vi "OCV Histogram gRPC.vi"() -> (1 "mean values of channels":dbl[](array[numeric]), 2 "std dev":dbl, 3 "range":dbl)   [LabVIEW 2019] (continued)
  in  "OCVResults 200Hz":T1[](array[typedef])=[{"battery1voltage"=3.4816475, "battery2voltage"=3.4830532, "battery3voltage"=3.4783754, "battery4voltage"=3.4823782, "battery5voltage"=3.4844217, "battery6voltage"=0.0, "battery7voltage"=0.0, "battery8voltage"=0.0, "battery9voltage"=0.0, "battery10voltage"=0.0, "battery11voltage"=0.0, "battery12voltage"=0.0, "battery13voltage"=0.0, "battery14voltage"=0.0, "battery15voltage"=0.0, "battery16voltage"=0.0, "battery17voltage"=0.0, "battery18voltage"=0.0, "battery19voltage"=0.0, "battery20voltage"=0.0, "battery21voltage"=0.0, "battery22voltage"=0.0, "battery23voltage"=0.0, "battery24voltage"=0.0, "ErrorOutData"={"ErrorCode"=0, "ErrorMessage"=""}}, {"battery1voltage"=3.4816465, "battery2voltage"=3.4830518, "battery3voltage"=3.4783754, "battery4voltage"=3.4823792, "battery5voltage"=3.484419, "battery6voltage"=0.0, "battery7voltage"=0.0, "battery8voltage"=0.0, "battery9voltage"=0.0, "battery10voltage"=0.0, "battery11voltage"=0.0, "battery12voltage"=0.0, "battery13voltage"=0.0, "battery14voltage"=0.0, "battery15voltage"=0.0, "battery16voltage"=0.0, "battery17voltage"=0.0, "battery18voltage"=0.0, "battery19voltage"=0.0, "battery20voltage"=0.0, "battery21voltage"=0.0, "battery22voltage"=0.0, "battery23voltage"=0.0, "battery24voltage"=0.0, "ErrorOutData"={"ErrorCode"=0, "ErrorMessage"=""}}, {"battery1voltage"=3.4816508, "battery2voltage"=3.483053, "battery3voltage"=3.4783792, "battery4voltage"=3.482379, "battery5voltage"=3.484414, "battery6voltage"=0.0, "battery7voltage"=0.0, "battery8voltage"=0.0, "battery9voltage"=0.0, "battery10voltage"=0.0, "battery11voltage"=0.0, "battery12voltage"=0.0, "battery13voltage"=0.0, "battery14voltage"=0.0, "battery15voltage"=0.0, "battery16voltage"=0.0, "battery17voltage"=0.0, "battery18voltage"=0.0, "battery19voltage"=0.0, "battery20voltage"=0.0, "battery21voltage"=0.0, "battery22voltage"=0.0, "battery23voltage"=0.0, "battery24voltage"=0.0, "ErrorOutData"={"ErrorCode"=0, "ErrorMessage"=""}}, {"battery1voltage"=3.4816496, "battery2voltage"=3.4830558, "battery3voltage"=3.4783785, "battery4voltage"=3.4823782, "battery5voltage"=3.484414, "battery6voltage"=0.0, "battery7voltage"=0.0, "battery8voltage"=0.0, "battery9voltage"=0.0, "battery10voltage"=0.0, "battery11voltage"=0.0, "battery12voltage"=0.0, "battery13voltage"=0.0, "battery14voltage"=0.0, "battery15voltage"=0.0, "battery16voltage"=0.0, "battery17voltage"=0.0, "battery18voltage"=0.0, "battery19voltage"=0.0, "battery20voltage"=0.0, "battery21voltage"=0.0, "battery22voltage"=0.0, "battery23voltage"=0.0, "battery24voltage"=0.0, "ErrorOutData"={"ErrorCode"=0, "ErrorMessage"=""}}, {"battery1voltage"=3.481646, "battery2voltage"=3.4830523, "battery3voltage"=3.4783762, "battery4voltage"=3.482376, "battery5voltage"=3.4844196, "battery6voltage"=0.0, "battery7voltage"=0.0, "battery8voltage"=0.0, "battery9voltage"=0.0, "battery10voltage"=0.0, "battery11voltage"=0.0, "battery12voltage"=0.0, "battery13voltage"=0.0, "battery14voltage"=0.0, "battery15voltage"=0.0, "battery16voltage"=0.0, "battery17voltage"=0.0, "battery18voltage"=0.0, "battery19voltage"=0.0, "battery20voltage"=0.0, "battery21voltage"=0.0, "battery22voltage"=0.0, "battery23voltage"=0.0, "battery24voltage"=0.0, "ErrorOutData"={"ErrorCode"=0, "ErrorMessage"=""}}, {"battery1voltage"=3.481651, "battery2voltage"=3.4830537, "battery3voltage"=3.4783807, "battery4voltage"=3.4823775, "battery5voltage"=3.484415, "battery6voltage"=0.0, "battery7voltage"=0.0, "battery8voltage"=0.0, "battery9voltage"=0.0, "battery10voltage"=0.0, "battery11voltage"=0.0, "battery12voltage"=0.0, "battery13voltage"=0.0, "battery14voltage"=0.0, "battery15voltage"=0.0, "battery16voltage"=0.0, "battery17voltage"=0.0, "battery18voltage"=0.0, "battery19voltage"=0.0, "battery20voltage"=0.0, "battery21voltage"=0.0, "battery22voltage"=0.0, "battery23voltage"=0.0, "battery24voltage"=0.0, "ErrorOutData"={"ErrorCode"=0, "ErrorMessage"=""}}, {"battery1voltage"=3.4816496, "battery2voltage"=3.4830575, "battery3voltage"=3.4783802, "battery4voltage"=3.4823804, "battery5voltage"=3.4844165, "battery6voltage"=0.0, "battery7voltage"=0.0, "battery8voltage"=0.0, "battery9voltage"=0.0, "battery10voltage"=0.0, "battery11voltage"=0.0, "battery12voltage"=0.0, "battery13voltage"=0.0, "battery14voltage"=0.0, "battery15voltage"=0.0, "battery16voltage"=0.0, "battery17voltage"=0.0, "battery18voltage"=0.0, "battery19voltage"=0.0, "battery20voltage"=0.0, "battery21voltage"=0.0, "battery22voltage"=0.0, "battery23voltage"=0.0, "battery24voltage"=0.0, "ErrorOutData"={"ErrorCode"=0, "ErrorMessage"=""}}, {"battery1voltage"=3.4816468, "battery2voltage"=3.4830506, "battery3voltage"=3.4783757, "battery4voltage"=3.4823778, "battery5voltage"=3.484419, "battery6voltage"=0.0, "battery7voltage"=0.0, "battery8voltage"=0.0, "battery9voltage"=0.0, "battery10voltage"=0.0, "battery11voltage"=0.0, "battery12voltage"=0.0, "battery13voltage"=0.0, "battery14voltage"=0.0, "battery15voltage"=0.0, "battery16voltage"=0.0, "battery17voltage"=0.0, "battery18voltage"=0.0, "battery19voltage"=0.0, "battery20voltage"=0.0, "battery21voltage"=0.0, "battery22voltage"=0.0, "battery23voltage"=0.0, "battery24voltage"=0.0, "ErrorOutData"={"ErrorCode"=0, "ErrorMessage"=""}}, {"battery1voltage"=3.4816494, "battery2voltage"=3.4830542, "battery3voltage"=3.4783788, "battery4voltage"=3.4823797, "battery5voltage"=3.4844136, "battery6voltage"=0.0, "battery7voltage"=0.0, "battery8voltage"=0.0, "battery9voltage"=0.0, "battery10voltage"=0.0, "battery11voltage"=0.0, "battery12voltage"=0.0, "battery13voltage"=0.0, "battery14voltage"=0.0, "battery15voltage"=0.0, "battery16voltage"=0.0, "battery17voltage"=0.0, "battery18voltage"=0.0, "battery19voltage"=0.0, "battery20voltage"=0.0, "battery21voltage"=0.0, "battery22voltage"=0.0, "battery23voltage"=0.0, "battery24voltage"=0.0, "ErrorOutData"={"ErrorCode"=0, "ErrorMessage"=""}}, {"battery1voltage"=3.4816506, "battery2voltage"=3.483054, "battery3voltage"=3.4783807, "battery4voltage"=3.4823804, "battery5voltage"=3.4844153, "battery6voltage"=0.0, "battery7voltage"=0.0, "battery8voltage"=0.0, "battery9voltage"=0.0, "battery10voltage"=0.0, "battery11voltage"=0.0, "battery12voltage"=0.0, "battery13voltage"=0.0, "battery14voltage"=0.0, "battery15voltage"=0.0, "battery16voltage"=0.0, "battery17voltage"=0.0, "battery18voltage"=0.0, "battery19voltage"=0.0, "battery20voltage"=0.0, "battery21voltage"=0.0, "battery22voltage"=0.0, "battery23voltage"=0.0, "battery24voltage"=0.0, "ErrorOutData"={"ErrorCode"=0, "ErrorMessage"=""}}, {"battery1voltage"=3.481649, "battery2voltage"=3.4830494, "battery3voltage"=3.478376, "battery4voltage"=3.482376, "battery5voltage"=3.4844186, "battery6voltage"=0.0, "battery7voltage"=0.0, "battery8voltage"=0.0, "battery9voltage"=0.0, "battery10voltage"=0.0, "battery11voltage"=0.0, "battery12voltage"=0.0, "battery13voltage"=0.0, "battery14voltage"=0.0, "battery15voltage"=0.0, "battery16voltage"=0.0, "battery17voltage"=0.0, "battery18voltage"=0.0, "battery19voltage"=0.0, "battery20voltage"=0.0, "battery21voltage"=0.0, "battery22voltage"=0.0, "battery23voltage"=0.0, "battery24voltage"=0.0, "ErrorOutData"={"ErrorCode"=0, "ErrorMessage"=""}}, {"battery1voltage"=3.4816506, "battery2voltage"=3.483054, "battery3voltage"=3.4783802, "battery4voltage"=3.4823794, "battery5voltage"=3.4844139, "battery6voltage"=0.0, "battery7voltage"=0.0, "battery8voltage"=0.0, "battery9voltage"=0.0, "battery10voltage"=0.0, "battery11voltage"=0.0, "battery12voltage"=0.0, "battery13voltage"=0.0, "battery14voltage"=0.0, "battery15voltage"=0.0, "battery16voltage"=0.0, "battery17voltage"=0.0, "battery18voltage"=0.0, "battery19voltage"=0.0, "battery20voltage"=0.0, "battery21voltage"=0.0, "battery22voltage"=0.0, "battery23voltage"=0.0, "battery24voltage"=0.0, "ErrorOutData"={"ErrorCode"=0, "ErrorMessage"=""}}, {"battery1voltage"=3.481648, "battery2voltage"=3.483055, "battery3voltage"=3.4783783, "battery4voltage"=3.482379, "battery5voltage"=3.484413, "battery6voltage"=0.0, "battery7voltage"=0.0, "battery8voltage"=0.0, "battery9voltage"=0.0, "battery10voltage"=0.0, "battery11voltage"=0.0, "battery12voltage"=0.0, "battery13voltage"=0.0, "battery14voltage"=0.0, "battery15voltage"=0.0, "battery16voltage"=0.0, "battery17voltage"=0.0, "battery18voltage"=0.0, "battery19voltage"=0.0, "battery20voltage"=0.0, "battery21voltage"=0.0, "battery22voltage"=0.0, "battery23voltage"=0.0, "battery24voltage"=0.0, "ErrorOutData"={"ErrorCode"=0, "ErrorMessage"=""}}, {"battery1voltage"=3.4816458, "battery2voltage"=3.483052, "battery3voltage"=3.4783766, "battery4voltage"=3.4823794, "battery5voltage"=3.484419, "battery6voltage"=0.0, "battery7voltage"=0.0, "battery8voltage"=0.0, "battery9voltage"=0.0, "battery10voltage"=0.0, "battery11voltage"=0.0, "battery12voltage"=0.0, "battery13voltage"=0.0, "battery14voltage"=0.0, "battery15voltage"=0.0, "battery16voltage"=0.0, "battery17voltage"=0.0, "battery18voltage"=0.0, "battery19voltage"=0.0, "battery20voltage"=0.0, "battery21voltage"=0.0, "battery22voltage"=0.0, "battery23voltage"=0.0, "battery24voltage"=0.0, "ErrorOutData"={"ErrorCode"=0, "ErrorMessage"=""}}, {"battery1voltage"=3.4816475, "battery2voltage"=3.4830542, "battery3voltage"=3.4783762, "battery4voltage"=3.482376, "battery5voltage"=3.484421, "battery6voltage"=0.0, "battery7voltage"=0.0, "battery8voltage"=0.0, "battery9voltage"=0.0, "battery10voltage"=0.0, "battery11voltage"=0.0, "battery12voltage"=0.0, "battery13voltage"=0.0, "battery14voltage"=0.0, "battery15voltage"=0.0, "battery16voltage"=0.0, "battery17voltage"=0.0, "battery18voltage"=0.0, "battery19voltage"=0.0, "battery20voltage"=0.0, "battery21voltage"=0.0, "battery22voltage"=0.0, "battery23voltage"=0.0, "battery24voltage"=0.0, "ErrorOutData"={"ErrorCode"=0, "ErrorMessage"=""}}, {"battery1voltage"=3.4816487, "battery2voltage"=3.4830506, "battery3voltage"=3.4783754, "battery4voltage"=3.482377, "battery5voltage"=3.4844167, "battery6voltage"=0.0, "battery7voltage"=0.0, "battery8voltage"=0.0, "battery9voltage"=0.0, "battery10voltage"=0.0, "battery11voltage"=0.0, "battery12voltage"=0.0, "battery13voltage"=0.0, "battery14voltage"=0.0, "battery15voltage"=0.0, "battery16voltage"=0.0, "battery17voltage"=0.0, "battery18voltage"=0.0, "battery19voltage"=0.0, "battery20voltage"=0.0, "battery21voltage"=0.0, "battery22voltage"=0.0, "battery23voltage"=0.0, "battery24voltage"=0.0, "ErrorOutData"={"ErrorCode"=0, "ErrorMessage"=""}}, {"battery1voltage"=3.4816504, "battery2voltage"=3.483053, "battery3voltage"=3.4783785, "battery4voltage"=3.4823782, "battery5voltage"=3.4844148, "battery6voltage"=0.0, "battery7voltage"=0.0, "battery8voltage"=0.0, "battery9voltage"=0.0, "battery10voltage"=0.0, "battery11voltage"=0.0, "battery12voltage"=0.0, "battery13voltage"=0.0, "battery14voltage"=0.0, "battery15voltage"=0.0, "battery16voltage"=0.0, "battery17voltage"=0.0, "battery18voltage"=0.0, "battery19voltage"=0.0, "battery20voltage"=0.0, "battery21voltage"=0.0, "battery22voltage"=0.0, "battery23voltage"=0.0, "battery24voltage"=0.0, "ErrorOutData"={"ErrorCode"=0, "ErrorMessage"=""}}, {"battery1voltage"=3.4816487, "battery2voltage"=3.4830518, "battery3voltage"=3.4783754, "battery4voltage"=3.482377, "battery5voltage"=3.4844203, "battery6voltage"=0.0, "battery7voltage"=0.0, "battery8voltage"=0.0, "battery9voltage"=0.0, "battery10voltage"=0.0, "battery11voltage"=0.0, "battery12voltage"=0.0, "battery13voltage"=0.0, "battery14voltage"=0.0, "battery15voltage"=0.0, "battery16voltage"=0.0, "battery17voltage"=0.0, "battery18voltage"=0.0, "battery19voltage"=0.0, "battery20voltage"=0.0, "battery21voltage"=0.0, "battery22voltage"=0.0, "battery23voltage"=0.0, "battery24voltage"=0.0, "ErrorOutData"={"ErrorCode"=0, "ErrorMessage"=""}}, {"battery1voltage"=3.4816482, "battery2voltage"=3.4830515, "battery3voltage"=3.4783762, "battery4voltage"=3.4823794, "battery5voltage"=3.484422, "battery6voltage"=0.0, "battery7voltage"=0.0, "battery8voltage"=0.0, "battery9voltage"=0.0, "battery10voltage"=0.0, "battery11voltage"=0.0, "battery12voltage"=0.0, "battery13voltage"=0.0, "battery14voltage"=0.0, "battery15voltage"=0.0, "battery16voltage"=0.0, "battery17voltage"=0.0, "battery18voltage"=0.0, "battery19voltage"=0.0, "battery20voltage"=0.0, "battery21voltage"=0.0, "battery22voltage"=0.0, "battery23voltage"=0.0, "battery24voltage"=0.0, "ErrorOutData"={"ErrorCode"=0, "ErrorMessage"=""}}, {"battery1voltage"=3.4816468, "battery2voltage"=3.4830506, "battery3voltage"=3.478376, "battery4voltage"=3.4823782, "battery5voltage"=3.484421, "battery6voltage"=0.0, "battery7voltage"=0.0, "battery8voltage"=0.0, "battery9voltage"=0.0, "battery10voltage"=0.0, "battery11voltage"=0.0, "battery12voltage"=0.0, "battery13voltage"=0.0, "battery14voltage"=0.0, "battery15voltage"=0.0, "battery16voltage"=0.0, "battery17voltage"=0.0, "battery18voltage"=0.0, "battery19voltage"=0.0, "battery20voltage"=0.0, "battery21voltage"=0.0, "battery22voltage"=0.0, "battery23voltage"=0.0, "battery24voltage"=0.0, "ErrorOutData"={"ErrorCode"=0, "ErrorMessage"=""}}, {"battery1voltage"=3.4816484, "battery2voltage"=3.4830525, "battery3voltage"=3.4783764, "battery4voltage"=3.4823756, "battery5voltage"=3.4844203, "battery6voltage"=0.0, "battery7voltage"=0.0, "battery8voltage"=0.0, "battery9voltage"=0.0, "battery10voltage"=0.0, "battery11voltage"=0.0, "battery12voltage"=0.0, "battery13voltage"=0.0, "battery14voltage"=0.0, "battery15voltage"=0.0, "battery16voltage"=0.0, "battery17voltage"=0.0, "battery18voltage"=0.0, "battery19voltage"=0.0, "battery20voltage"=0.0, "battery21voltage"=0.0, "battery22voltage"=0.0, "battery23voltage"=0.0, "battery24voltage"=0.0, "ErrorOutData"={"ErrorCode"=0, "ErrorMessage"=""}}, {"battery1voltage"=3.4816477, "battery2voltage"=3.4830525, "battery3voltage"=3.4783745, "battery4voltage"=3.482378, "battery5voltage"=3.484421, "battery6voltage"=0.0, "battery7voltage"=0.0, "battery8voltage"=0.0, "battery9voltage"=0.0, "battery10voltage"=0.0, "battery11voltage"=0.0, "battery12voltage"=0.0, "battery13voltage"=0.0, "battery14voltage"=0.0, "battery15voltage"=0.0, "battery16voltage"=0.0, "battery17voltage"=0.0, "battery18voltage"=0.0, "battery19voltage"=0.0, "battery20voltage"=0.0, "battery21voltage"=0.0, "battery22voltage"=0.0, "battery23voltage"=0.0, "battery24voltage"=0.0, "ErrorOutData"={"ErrorCode"=0, "ErrorMessage"=""}}, {"battery1voltage"=3.4816477, "battery2voltage"=3.4830518, "battery3voltage"=3.4783752, "battery4voltage"=3.4823785, "battery5voltage"=3.4844203, "battery6voltage"=0.0, "battery7voltage"=0.0, "battery8voltage"=0.0, "battery9voltage"=0.0, "battery10voltage"=0.0, "battery11voltage"=0.0, "battery12voltage"=0.0, "battery13voltage"=0.0, "battery14voltage"=0.0, "battery15voltage"=0.0, "battery16voltage"=0.0, "battery17voltage"=0.0, "battery18voltage"=0.0, "battery19voltage"=0.0, "battery20voltage"=0.0, "battery21voltage"=0.0, "battery22voltage"=0.0, "battery23voltage"=0.0, "battery24voltage"=0.0, "ErrorOutData"={"ErrorCode"=0, "ErrorMessage"=""}}, {"battery1voltage"=3.4816518, "battery2voltage"=3.4830563, "battery3voltage"=3.47838, "battery4voltage"=3.4823773, "battery5voltage"=3.4844139, "battery6voltage"=0.0, "battery7voltage"=0.0, "battery8voltage"=0.0, "battery9voltage"=0.0, "battery10voltage"=0.0, "battery11voltage"=0.0, "battery12voltage"=0.0, "battery13voltage"=0.0, "battery14voltage"=0.0, "battery15voltage"=0.0, "battery16voltage"=0.0, "battery17voltage"=0.0, "battery18voltage"=0.0, "battery19voltage"=0.0, "battery20voltage"=0.0, "battery21voltage"=0.0, "battery22voltage"=0.0, "battery23voltage"=0.0, "battery24voltage"=0.0, "ErrorOutData"={"ErrorCode"=0, "ErrorMessage"=""}}, {"battery1voltage"=3.4816487, "battery2voltage"=3.483055, "battery3voltage"=3.478379, "battery4voltage"=3.4823766, "battery5voltage"=3.484415, "battery6voltage"=0.0, "battery7voltage"=0.0, "battery8voltage"=0.0, "battery9voltage"=0.0, "battery10voltage"=0.0, "battery11voltage"=0.0, "battery12voltage"=0.0, "battery13voltage"=0.0, "battery14voltage"=0.0, "battery15voltage"=0.0, "battery16voltage"=0.0, "battery17voltage"=0.0, "battery18voltage"=0.0, "battery19voltage"=0.0, "battery20voltage"=0.0, "battery21voltage"=0.0, "battery22voltage"=0.0, "battery23voltage"=0.0, "battery24voltage"=0.0, "ErrorOutData"={"ErrorCode"=0, "ErrorMessage"=""}}, {"battery1voltage"=3.4816518, "battery2voltage"=3.483055, "battery3voltage"=3.4783797, "battery4voltage"=3.4823785, "battery5voltage"=3.4844165, "battery6voltage"=0.0, "battery7voltage"=0.0, "battery8voltage"=0.0, "battery9voltage"=0.0, "battery10voltage"=0.0, "battery11voltage"=0.0, "battery12voltage"=0.0, "battery13voltage"=0.0, "battery14voltage"=0.0, "battery15voltage"=0.0, "battery16voltage"=0.0, "battery17voltage"=0.0, "battery18voltage"=0.0, "battery19voltage"=0.0, "battery20voltage"=0.0, "battery21voltage"=0.0, "battery22voltage"=0.0, "battery23voltage"=0.0, "battery24voltage"=0.0, "ErrorOutData"={"ErrorCode"=0, "ErrorMessage"=""}}, {"battery1voltage"=3.481648, "battery2voltage"=3.4830523, "battery3voltage"=3.4783738, "battery4voltage"=3.4823773, "battery5voltage"=3.48442, "battery6voltage"=0.0, "battery7voltage"=0.0, "battery8voltage"=0.0, "battery9voltage"=0.0, "battery10voltage"=0.0, "battery11voltage"=0.0, "battery12voltage"=0.0, "battery13voltage"=0.0, "battery14voltage"=0.0, "battery15voltage"=0.0, "battery16voltage"=0.0, "battery17voltage"=0.0, "battery18voltage"=0.0, "battery19voltage"=0.0, "battery20voltage"=0.0, "battery21voltage"=0.0, "battery22voltage"=0.0, "battery23voltage"=0.0, "battery24voltage"=0.0, "ErrorOutData"={"ErrorCode"=0, "ErrorMessage"=""}}, {"battery1voltage"=3.481649, "battery2voltage"=3.4830487, "battery3voltage"=3.4783742, "battery4voltage"=3.482377, "battery5voltage"=3.484417, "battery6voltage"=0.0, "battery7voltage"=0.0, "battery8voltage"=0.0, "battery9voltage"=0.0, "battery10voltage"=0.0, "battery11voltage"=0.0, "battery12voltage"=0.0, "battery13voltage"=0.0, "battery14voltage"=0.0, "battery15voltage"=0.0, "battery16voltage"=0.0, "battery17voltage"=0.0, "battery18voltage"=0.0, "battery19voltage"=0.0, "battery20voltage"=0.0, "battery21voltage"=0.0, "battery22voltage"=0.0, "battery23voltage"=0.0, "battery24voltage"=0.0, "ErrorOutData"={"ErrorCode"=0, "ErrorMessage"=""}}, {"battery1voltage"=3.4816473, "battery2voltage"=3.4830534, "battery3voltage"=3.4783776, "battery4voltage"=3.4823763, "battery5voltage"=3.4844205, "battery6voltage"=0.0, "battery7voltage"=0.0, "battery8voltage"=0.0, "battery9voltage"=0.0, "battery10voltage"=0.0, "battery11voltage"=0.0, "battery12voltage"=0.0, "battery13voltage"=0.0, "battery14voltage"=0.0, "battery15voltage"=0.0, "battery16voltage"=0.0, "battery17voltage"=0.0, "battery18voltage"=0.0, "battery19voltage"=0.0, "battery20voltage"=0.0, "battery21voltage"=0.0, "battery22voltage"=0.0, "battery23voltage"=0.0, "battery24voltage"=0.0, "ErrorOutData"={"ErrorCode"=0, "ErrorMessage"=""}}, {"battery1voltage"=3.4816482, "battery2voltage"=3.4830527, "battery3voltage"=3.4783754, "battery4voltage"=3.482379, "battery5voltage"=3.4844193, "battery6voltage"=0.0, "battery7voltage"=0.0, "battery8voltage"=0.0, "battery9voltage"=0.0, "battery10voltage"=0.0, "battery11voltage"=0.0, "battery12voltage"=0.0, "battery13voltage"=0.0, "battery14voltage"=0.0, "battery15voltage"=0.0, "battery16voltage"=0.0, "battery17voltage"=0.0, "battery18voltage"=0.0, "battery19voltage"=0.0, "battery20voltage"=0.0, "battery21voltage"=0.0, "battery22voltage"=0.0, "battery23voltage"=0.0, "battery24voltage"=0.0, "ErrorOutData"={"ErrorCode"=0, "ErrorMessage"=""}}, {"battery1voltage"=3.4816475, "battery2voltage"=3.4830527, "battery3voltage"=3.4783762, "battery4voltage"=3.4823744, "battery5voltage"=3.4844196, "battery6voltage"=0.0, "battery7voltage"=0.0, "battery8voltage"=0.0, "battery9voltage"=0.0, "battery10voltage"=0.0, "battery11voltage"=0.0, "battery12voltage"=0.0, "battery13voltage"=0.0, "battery14voltage"=0.0, "battery15voltage"=0.0, "battery16voltage"=0.0, "battery17voltage"=0.0, "battery18voltage"=0.0, "battery19voltage"=0.0, "battery20voltage"=0.0, "battery21voltage"=0.0, "battery22voltage"=0.0, "battery23voltage"=0.0, "battery24voltage"=0.0, "ErrorOutData"={"ErrorCode"=0, "ErrorMessage"=""}}, {"battery1voltage"=3.4816487, "battery2voltage"=3.4830544, "battery3voltage"=3.478379, "battery4voltage"=3.4823763, "battery5voltage"=3.4844158, "battery6voltage"=0.0, "battery7voltage"=0.0, "battery8voltage"=0.0, "battery9voltage"=0.0, "battery10voltage"=0.0, "battery11voltage"=0.0, "battery12voltage"=0.0, "battery13voltage"=0.0, "battery14voltage"=0.0, "battery15voltage"=0.0, "battery16voltage"=0.0, "battery17voltage"=0.0, "battery18voltage"=0.0, "battery19voltage"=0.0, "battery20voltage"=0.0, "battery21voltage"=0.0, "battery22voltage"=0.0, "battery23voltage"=0.0, "battery24voltage"=0.0, "ErrorOutData"={"ErrorCode"=0, "ErrorMessage"=""}}, {"battery1voltage"=3.481652, "battery2voltage"=3.4830534, "battery3voltage"=3.4783797, "battery4voltage"=3.4823794, "battery5voltage"=3.4844155, "battery6voltage"=0.0, "battery7voltage"=0.0, "battery8voltage"=0.0, "battery9voltage"=0.0, "battery10voltage"=0.0, "battery11voltage"=0.0, "battery12voltage"=0.0, "battery13voltage"=0.0, "battery14voltage"=0.0, "battery15voltage"=0.0, "battery16voltage"=0.0, "battery17voltage"=0.0, "battery18voltage"=0.0, "battery19voltage"=0.0, "battery20voltage"=0.0, "battery21voltage"=0.0, "battery22voltage"=0.0, "battery23voltage"=0.0, "battery24voltage"=0.0, "ErrorOutData"={"ErrorCode"=0, "ErrorMessage"=""}}, {"battery1voltage"=3.481647, "battery2voltage"=3.483051, "battery3voltage"=3.4783762, "battery4voltage"=3.4823768, "battery5voltage"=3.4844208, "battery6voltage"=0.0, "battery7voltage"=0.0, "battery8voltage"=0.0, "battery9voltage"=0.0, "battery10voltage"=0.0, "battery11voltage"=0.0, "battery12voltage"=0.0, "battery13voltage"=0.0, "battery14voltage"=0.0, "battery15voltage"=0.0, "battery16voltage"=0.0, "battery17voltage"=0.0, "battery18voltage"=0.0, "battery19voltage"=0.0, "battery20voltage"=0.0, "battery21voltage"=0.0, "battery22voltage"=0.0, "battery23voltage"=0.0, "battery24voltage"=0.0, "ErrorOutData"={"ErrorCode"=0, "ErrorMessage"=""}}, {"battery1voltage"=3.481646, "battery2voltage"=3.4830496, "battery3voltage"=3.4783783, "battery4voltage"=3.4823778, "battery5voltage"=3.4844189, "battery6voltage"=0.0, "battery7voltage"=0.0, "battery8voltage"=0.0, "battery9voltage"=0.0, "battery10voltage"=0.0, "battery11voltage"=0.0, "battery12voltage"=0.0, "battery13voltage"=0.0, "battery14voltage"=0.0, "battery15voltage"=0.0, "battery16voltage"=0.0, "battery17voltage"=0.0, "battery18voltage"=0.0, "battery19voltage"=0.0, "battery20voltage"=0.0, "battery21voltage"=0.0, "battery22voltage"=0.0, "battery23voltage"=0.0, "battery24voltage"=0.0, "ErrorOutData"={"ErrorCode"=0, "ErrorMessage"=""}}, {"battery1voltage"=3.4816482, "battery2voltage"=3.4830515, "battery3voltage"=3.4783747, "battery4voltage"=3.4823802, "battery5voltage"=3.484419, "battery6voltage"=0.0, "battery7voltage"=0.0, "battery8voltage"=0.0, "battery9voltage"=0.0, "battery10voltage"=0.0, "battery11voltage"=0.0, "battery12voltage"=0.0, "battery13voltage"=0.0, "battery14voltage"=0.0, "battery15voltage"=0.0, "battery16voltage"=0.0, "battery17voltage"=0.0, "battery18voltage"=0.0, "battery19voltage"=0.0, "battery20voltage"=0.0, "battery21voltage"=0.0, "battery22voltage"=0.0, "battery23voltage"=0.0, "battery24voltage"=0.0, "ErrorOutData"={"ErrorCode"=0, "ErrorMessage"=""}}, {"battery1voltage"=3.4816465, "battery2voltage"=3.48305, "battery3voltage"=3.4783783, "battery4voltage"=3.4823782, "battery5voltage"=3.4844184, "battery6voltage"=0.0, "battery7voltage"=0.0, "battery8voltage"=0.0, "battery9voltage"=0.0, "battery10voltage"=0.0, "battery11voltage"=0.0, "battery12voltage"=0.0, "battery13voltage"=0.0, "battery14voltage"=0.0, "battery15voltage"=0.0, "battery16voltage"=0.0, "battery17voltage"=0.0, "battery18voltage"=0.0, "battery19voltage"=0.0, "battery20voltage"=0.0, "battery21voltage"=0.0, "battery22voltage"=0.0, "battery23voltage"=0.0, "battery24voltage"=0.0, "ErrorOutData"={"ErrorCode"=0, "ErrorMessage"=""}}, {"battery1voltage"=3.481649, "battery2voltage"=3.4830534, "battery3voltage"=3.4783783, "battery4voltage"=3.4823785, "battery5voltage"=3.4844139, "battery6voltage"=0.0, "battery7voltage"=0.0, "battery8voltage"=0.0, "battery9voltage"=0.0, "battery10voltage"=0.0, "battery11voltage"=0.0, "battery12voltage"=0.0, "battery13voltage"=0.0, "battery14voltage"=0.0, "battery15voltage"=0.0, "battery16voltage"=0.0, "battery17voltage"=0.0, "battery18voltage"=0.0, "battery19voltage"=0.0, "battery20voltage"=0.0, "battery21voltage"=0.0, "battery22voltage"=0.0, "battery23voltage"=0.0, "battery24voltage"=0.0, "ErrorOutData"={"ErrorCode"=0, "ErrorMessage"=""}}, {"battery1voltage"=3.4816468, "battery2voltage"=3.483055, "battery3voltage"=3.4783797, "battery4voltage"=3.4823809, "battery5voltage"=3.4844143, "battery6voltage"=0.0, "battery7voltage"=0.0, "battery8voltage"=0.0, "battery9voltage"=0.0, "battery10voltage"=0.0, "battery11voltage"=0.0, "battery12voltage"=0.0, "battery13voltage"=0.0, "battery14voltage"=0.0, "battery15voltage"=0.0, "battery16voltage"=0.0, "battery17voltage"=0.0, "battery18voltage"=0.0, "battery19voltage"=0.0, "battery20voltage"=0.0, "battery21voltage"=0.0, "battery22voltage"=0.0, "battery23voltage"=0.0, "battery24voltage"=0.0, "ErrorOutData"={"ErrorCode"=0, "ErrorMessage"=""}}, {"battery1voltage"=3.4816508, "battery2voltage"=3.4830515, "battery3voltage"=3.4783788, "battery4voltage"=3.4823782, "battery5voltage"=3.4844167, "battery6voltage"=0.0, "battery7voltage"=0.0, "battery8voltage"=0.0, "battery9voltage"=0.0, "battery10voltage"=0.0, "battery11voltage"=0.0, "battery12voltage"=0.0, "battery13voltage"=0.0, "battery14voltage"=0.0, "battery15voltage"=0.0, "battery16voltage"=0.0, "battery17voltage"=0.0, "battery18voltage"=0.0, "battery19voltage"=0.0, "battery20voltage"=0.0, "battery21voltage"=0.0, "battery22voltage"=0.0, "battery23voltage"=0.0, "battery24voltage"=0.0, "ErrorOutData"={"ErrorCode"=0, "ErrorMessage"=""}}, {"battery1voltage"=3.4816468, "battery2voltage"=3.4830503, "battery3voltage"=3.4783762, "battery4voltage"=3.4823782, "battery5voltage"=3.4844193, "battery6voltage"=0.0, "battery7voltage"=0.0, "battery8voltage"=0.0, "battery9voltage"=0.0, "battery10voltage"=0.0, "battery11voltage"=0.0, "battery12voltage"=0.0, "battery13voltage"=0.0, "battery14voltage"=0.0, "battery15voltage"=0.0, "battery16voltage"=0.0, "battery17voltage"=0.0, "battery18voltage"=0.0, "battery19voltage"=0.0, "battery20voltage"=0.0, "battery21voltage"=0.0, "battery22voltage"=0.0, "battery23voltage"=0.0, "battery24voltage"=0.0, "ErrorOutData"={"ErrorCode"=0, "ErrorMessage"=""}}, {"battery1voltage"=3.4816496, "battery2voltage"=3.4830527, "battery3voltage"=3.4783788, "battery4voltage"=3.482379, "battery5voltage"=3.484417, "battery6voltage"=0.0, "battery7voltage"=0.0, "battery8voltage"=0.0, "battery9voltage"=0.0, "battery10voltage"=0.0, "battery11voltage"=0.0, "battery12voltage"=0.0, "battery13voltage"=0.0, "battery14voltage"=0.0, "battery15voltage"=0.0, "battery16voltage"=0.0, "battery17voltage"=0.0, "battery18voltage"=0.0, "battery19voltage"=0.0, "battery20voltage"=0.0, "battery21voltage"=0.0, "battery22voltage"=0.0, "battery23voltage"=0.0, "battery24voltage"=0.0, "ErrorOutData"={"ErrorCode"=0, "ErrorMessage"=""}}, {"battery1voltage"=3.4816473, "battery2voltage"=3.4830494, "battery3voltage"=3.478376, "battery4voltage"=3.4823785, "battery5voltage"=3.4844203, "battery6voltage"=0.0, "battery7voltage"=0.0, "battery8voltage"=0.0, "battery9voltage"=0.0, "battery10voltage"=0.0, "battery11voltage"=0.0, "battery12voltage"=0.0, "battery13voltage"=0.0, "battery14voltage"=0.0, "battery15voltage"=0.0, "battery16voltage"=0.0, "battery17voltage"=0.0, "battery18voltage"=0.0, "battery19voltage"=0.0, "battery20voltage"=0.0, "battery21voltage"=0.0, "battery22voltage"=0.0, "battery23voltage"=0.0, "battery24voltage"=0.0, "ErrorOutData"={"ErrorCode"=0, "ErrorMessage"=""}}, {"battery1voltage"=3.4816525, "battery2voltage"=3.4830537, "battery3voltage"=3.4783804, "battery4voltage"=3.482377, "battery5voltage"=3.484416, "battery6voltage"=0.0, "battery7voltage"=0.0, "battery8voltage"=0.0, "battery9voltage"=0.0, "battery10voltage"=0.0, "battery11voltage"=0.0, "battery12voltage"=0.0, "battery13voltage"=0.0, "battery14voltage"=0.0, "battery15voltage"=0.0, "battery16voltage"=0.0, "battery17voltage"=0.0, "battery18voltage"=0.0, "battery19voltage"=0.0, "battery20voltage"=0.0, "battery21voltage"=0.0, "battery22voltage"=0.0, "battery23voltage"=0.0, "battery24voltage"=0.0, "ErrorOutData"={"ErrorCode"=0, "ErrorMessage"=""}}, {"battery1voltage"=3.4816463, "battery2voltage"=3.4830518, "battery3voltage"=3.478375, "battery4voltage"=3.4823782, "battery5voltage"=3.4844203, "battery6voltage"=0.0, "battery7voltage"=0.0, "battery8voltage"=0.0, "battery9voltage"=0.0, "battery10voltage"=0.0, "battery11voltage"=0.0, "battery12voltage"=0.0, "battery13voltage"=0.0, "battery14voltage"=0.0, "battery15voltage"=0.0, "battery16voltage"=0.0, "battery17voltage"=0.0, "battery18voltage"=0.0, "battery19voltage"=0.0, "battery20voltage"=0.0, "battery21voltage"=0.0, "battery22voltage"=0.0, "battery23voltage"=0.0, "battery24voltage"=0.0, "ErrorOutData"={"ErrorCode"=0, "ErrorMessage"=""}}, {"battery1voltage"=3.4816508, "battery2voltage"=3.4830534, "battery3voltage"=3.4783785, "battery4voltage"=3.4823804, "battery5voltage"=3.4844153, "battery6voltage"=0.0, "battery7voltage"=0.0, "battery8voltage"=0.0, "battery9voltage"=0.0, "battery10voltage"=0.0, "battery11voltage"=0.0, "battery12voltage"=0.0, "battery13voltage"=0.0, "battery14voltage"=0.0, "battery15voltage"=0.0, "battery16voltage"=0.0, "battery17voltage"=0.0, "battery18voltage"=0.0, "battery19voltage"=0.0, "battery20voltage"=0.0, "battery21voltage"=0.0, "battery22voltage"=0.0, "battery23voltage"=0.0, "battery24voltage"=0.0, "ErrorOutData"={"ErrorCode"=0, "ErrorMessage"=""}}, {"battery1voltage"=3.4816477, "battery2voltage"=3.4830525, "battery3voltage"=3.4783752, "battery4voltage"=3.4823787, "battery5voltage"=3.4844213, "battery6voltage"=0.0, "battery7voltage"=0.0, "battery8voltage"=0.0, "battery9voltage"=0.0, "battery10voltage"=0.0, "battery11voltage"=0.0, "battery12voltage"=0.0, "battery13voltage"=0.0, "battery14voltage"=0.0, "battery15voltage"=0.0, "battery16voltage"=0.0, "battery17voltage"=0.0, "battery18voltage"=0.0, "battery19voltage"=0.0, "battery20voltage"=0.0, "battery21voltage"=0.0, "battery22voltage"=0.0, "battery23voltage"=0.0, "battery24voltage"=0.0, "ErrorOutData"={"ErrorCode"=0, "ErrorMessage"=""}}, {"battery1voltage"=3.4816494, "battery2voltage"=3.4830534, "battery3voltage"=3.4783752, "battery4voltage"=3.4823754, "battery5voltage"=3.4844198, "battery6voltage"=0.0, "battery7voltage"=0.0, "battery8voltage"=0.0, "battery9voltage"=0.0, "battery10voltage"=0.0, "battery11voltage"=0.0, "battery12voltage"=0.0, "battery13voltage"=0.0, "battery14voltage"=0.0, "battery15voltage"=0.0, "battery16voltage"=0.0, "battery17voltage"=0.0, "battery18voltage"=0.0, "battery19voltage"=0.0, "battery20voltage"=0.0, "battery21voltage"=0.0, "battery22voltage"=0.0, "battery23voltage"=0.0, "battery24voltage"=0.0, "ErrorOutData"={"ErrorCode"=0, "ErrorMessage"=""}}, {"battery1voltage"=3.481651, "battery2voltage"=3.483054, "battery3voltage"=3.478381, "battery4voltage"=3.4823792, "battery5voltage"=3.484416, "battery6voltage"=0.0, "battery7voltage"=0.0, "battery8voltage"=0.0, "battery9voltage"=0.0, "battery10voltage"=0.0, "battery11voltage"=0.0, "battery12voltage"=0.0, "battery13voltage"=0.0, "battery14voltage"=0.0, "battery15voltage"=0.0, "battery16voltage"=0.0, "battery17voltage"=0.0, "battery18voltage"=0.0, "battery19voltage"=0.0, "battery20voltage"=0.0, "battery21voltage"=0.0, "battery22voltage"=0.0, "battery23voltage"=0.0, "battery24voltage"=0.0, "ErrorOutData"={"ErrorCode"=0, "ErrorMessage"=""}}, {"battery1voltage"=3.4816496, "battery2voltage"=3.4830537, "battery3voltage"=3.4783804, "battery4voltage"=3.4823782, "battery5voltage"=3.484416, "battery6voltage"=0.0, "battery7voltage"=0.0, "battery8voltage"=0.0, "battery9voltage"=0.0, "battery10voltage"=0.0, "battery11voltage"=0.0, "battery12voltage"=0.0, "battery13voltage"=0.0, "battery14voltage"=0.0, "battery15voltage"=0.0, "battery16voltage"=0.0, "battery17voltage"=0.0, "battery18voltage"=0.0, "battery19voltage"=0.0, "battery20voltage"=0.0, "battery21voltage"=0.0, "battery22voltage"=0.0, "battery23voltage"=0.0, "battery24voltage"=0.0, "ErrorOutData"={"ErrorCode"=0, "ErrorMessage"=""}}, {"battery1voltage"=3.4816473, "battery2voltage"=3.4830506, "battery3voltage"=3.478376, "battery4voltage"=3.4823792, "battery5voltage"=3.4844186, "battery6voltage"=0.0, "battery7voltage"=0.0, "battery8voltage"=0.0, "battery9voltage"=0.0, "battery10voltage"=0.0, "battery11voltage"=0.0, "battery12voltage"=0.0, "battery13voltage"=0.0, "battery14voltage"=0.0, "battery15voltage"=0.0, "battery16voltage"=0.0, "battery17voltage"=0.0, "battery18voltage"=0.0, "battery19voltage"=0.0, "battery20voltage"=0.0, "battery21voltage"=0.0, "battery22voltage"=0.0, "battery23voltage"=0.0, "battery24voltage"=0.0, "ErrorOutData"={"ErrorCode"=0, "ErrorMessage"=""}}, {"battery1voltage"=3.4816515, "battery2voltage"=3.4830534, "battery3voltage"=3.4783795, "battery4voltage"=3.4823778, "battery5voltage"=3.484414, "battery6voltage"=0.0, "battery7voltage"=0.0, "battery8voltage"=0.0, "battery9voltage"=0.0, "battery10voltage"=0.0, "battery11voltage"=0.0, "battery12voltage"=0.0, "battery13voltage"=0.0, "battery14voltage"=0.0, "battery15voltage"=0.0, "battery16voltage"=0.0, "battery17voltage"=0.0, "battery18voltage"=0.0, "battery19voltage"=0.0, "battery20voltage"=0.0, "battery21voltage"=0.0, "battery22voltage"=0.0, "battery23voltage"=0.0, "battery24voltage"=0.0, "ErrorOutData"={"ErrorCode"=0, "ErrorMessage"=""}}, {"battery1voltage"=3.4816475, "battery2voltage"=3.4830518, "battery3voltage"=3.4783747, "battery4voltage"=3.4823778, "battery5voltage"=3.4844196, "battery6voltage"=0.0, "battery7voltage"=0.0, "battery8voltage"=0.0, "battery9voltage"=0.0, "battery10voltage"=0.0, "battery11voltage"=0.0, "battery12voltage"=0.0, "battery13voltage"=0.0, "battery14voltage"=0.0, "battery15voltage"=0.0, "battery16voltage"=0.0, "battery17voltage"=0.0, "battery18voltage"=0.0, "battery19voltage"=0.0, "battery20voltage"=0.0, "battery21voltage"=0.0, "battery22voltage"=0.0, "battery23voltage"=0.0, "battery24voltage"=0.0, "ErrorOutData"={"ErrorCode"=0, "ErrorMessage"=""}}, {"battery1voltage"=3.4816484, "battery2voltage"=3.4830515, "battery3voltage"=3.478376, "battery4voltage"=3.4823766, "battery5voltage"=3.4844193, "battery6voltage"=0.0, "battery7voltage"=0.0, "battery8voltage"=0.0, "battery9voltage"=0.0, "battery10voltage"=0.0, "battery11voltage"=0.0, "battery12voltage"=0.0, "battery13voltage"=0.0, "battery14voltage"=0.0, "battery15voltage"=0.0, "battery16voltage"=0.0, "battery17voltage"=0.0, "battery18voltage"=0.0, "battery19voltage"=0.0, "battery20voltage"=0.0, "battery21voltage"=0.0, "battery22voltage"=0.0, "battery23voltage"=0.0, "battery24voltage"=0.0, "ErrorOutData"={"ErrorCode"=0, "ErrorMessage"=""}}, {"battery1voltage"=3.481647, "battery2voltage"=3.4830508, "battery3voltage"=3.4783766, "battery4voltage"=3.4823794, "battery5voltage"=3.484418, "battery6voltage"=0.0, "battery7voltage"=0.0, "battery8voltage"=0.0, "battery9voltage"=0.0, "battery10voltage"=0.0, "battery11voltage"=0.0, "battery12voltage"=0.0, "battery13voltage"=0.0, "battery14voltage"=0.0, "battery15voltage"=0.0, "battery16voltage"=0.0, "battery17voltage"=0.0, "battery18voltage"=0.0, "battery19voltage"=0.0, "battery20voltage"=0.0, "battery21voltage"=0.0, "battery22voltage"=0.0, "battery23voltage"=0.0, "battery24voltage"=0.0, "ErrorOutData"={"ErrorCode"=0, "ErrorMessage"=""}}, {"battery1voltage"=3.4816504, "battery2voltage"=3.4830556, "battery3voltage"=3.4783795, "battery4voltage"=3.4823802, "battery5voltage"=3.4844158, "battery6voltage"=0.0, "battery7voltage"=0.0, "battery8voltage"=0.0, "battery9voltage"=0.0, "battery10voltage"=0.0, "battery11voltage"=0.0, "battery12voltage"=0.0, "battery13voltage"=0.0, "battery14voltage"=0.0, "battery15voltage"=0.0, "battery16voltage"=0.0, "battery17voltage"=0.0, "battery18voltage"=0.0, "battery19voltage"=0.0, "battery20voltage"=0.0, "battery21voltage"=0.0, "battery22voltage"=0.0, "battery23voltage"=0.0, "battery24voltage"=0.0, "ErrorOutData"={"ErrorCode"=0, "ErrorMessage"=""}}, {"battery1voltage"=3.4816482, "battery2voltage"=3.4830508, "battery3voltage"=3.478373, "battery4voltage"=3.4823759, "battery5voltage"=3.4844196, "battery6voltage"=0.0, "battery7voltage"=0.0, "battery8voltage"=0.0, "battery9voltage"=0.0, "battery10voltage"=0.0, "battery11voltage"=0.0, "battery12voltage"=0.0, "battery13voltage"=0.0, "battery14voltage"=0.0, "battery15voltage"=0.0, "battery16voltage"=0.0, "battery17voltage"=0.0, "battery18voltage"=0.0, "battery19voltage"=0.0, "battery20voltage"=0.0, "battery21voltage"=0.0, "battery22voltage"=0.0, "battery23voltage"=0.0, "battery24voltage"=0.0, "ErrorOutData"={"ErrorCode"=0, "ErrorMessage"=""}}, {"battery1voltage"=3.4816487, "battery2voltage"=3.4830518, "battery3voltage"=3.4783752, "battery4voltage"=3.4823768, "battery5voltage"=3.48442, "battery6voltage"=0.0, "battery7voltage"=0.0, "battery8voltage"=0.0, "battery9voltage"=0.0, "battery10voltage"=0.0, "battery11voltage"=0.0, "battery12voltage"=0.0, "battery13voltage"=0.0, "battery14voltage"=0.0, "battery15voltage"=0.0, "battery16voltage"=0.0, "battery17voltage"=0.0, "battery18voltage"=0.0, 
